vi "FGV - Acquisition Status.vi"(5 "mem loc":i32, 7 "Actions":T2=enum."Clear", 8 "Error In":errorcluster, 9 "Quit status":bool, 10 "Scan Type [In]":T1) -> (0 "Error Out":errorcluster, 1 "Quit status out":bool, 2 "Scan Type [Out]":T1, 4 "mem loc out":i32)   [LabVIEW 2018]
uses:
  Controls/FGV Actions.ctl
  Controls/ScanType.ctl
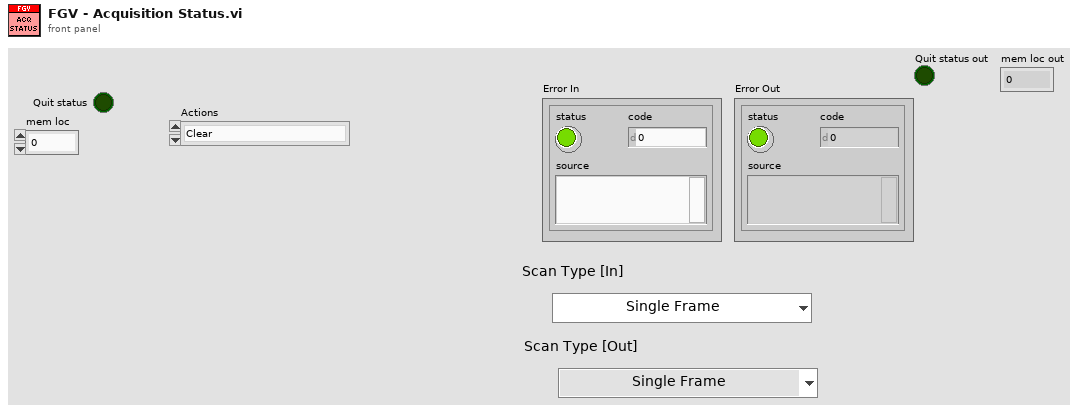
[diagram p1: front panel]
types:
  T1 = typedef "ScanType.ctl" = enum16{"Single Frame", "Continuous Frame", "ROI Line", "Vibratome", "Mosaic", "Mosaic + Slice"}
  T2 = typedef "FGV Actions.ctl" = enum16{"Init", "Set", "Get", "Clear"}
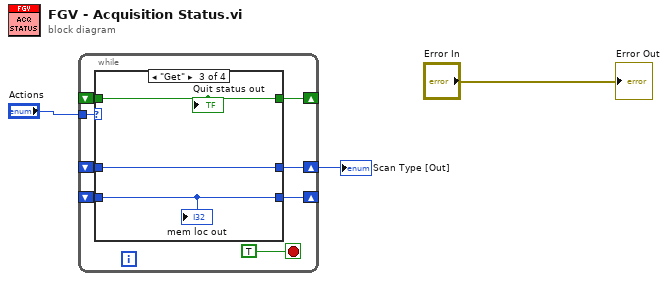
[diagram p0: block diagram]
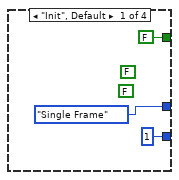
[diagram p2: hidden frame]
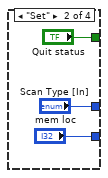
[diagram p3: hidden frame]
diagram:
  n1 = while {
    tunnel: "Actions" -> [w10]
    shift-right: [w9] -> w1
    shift-left: _ -> [w8]
    shift-right: [w7] -> _
    shift-left: _ -> [w6]
    shift-right: [w5] -> _
    shift-left: _ -> [w4]
    stop <- TRUE stop-if-true
    n2 = case shown="\"Get\"" w10 {
      tunnel: [ScanType."Single Frame" ("Scan Type") "Scan Type [In]" w20 _] -> w9
      tunnel: w8 -> [_ _ w20 _]
      tunnel: [FALSE ("Quit status") "Quit status" w19 _] -> w7
      tunnel: w6 -> [_ _ w19 _]
      tunnel: [1 ("mem loc") "mem loc" w18 _] -> w5
      tunnel: w4 -> [_ _ w18 _]
      frame "Init", Default {
        (unwired) FALSE
        (unwired) FALSE
      }
      frame "Set" {
      }
      frame "Get" {
        "Quit status out" <- w19
        "mem loc out" <- w18
      }
      frame "Clear" {
      }
    }
  }
  "Scan Type [Out]" <- w1
  "Error Out" <- "Error In"
